vi "List Available Tags.vi"(8 "error in (no error)":errorcluster, 10 "engine":refnum<data-value>, 11 "E2E editor node in":refnum<data-value>) -> (0 "error out":errorcluster, 1 "Available Tags":refnum<class "tag descriptor.lvclass">[](array[class]), 2 "engine out":refnum<data-value>, 3 "E2E editor node out":refnum<data-value>)   [LabVIEW 2015, in "E2E Tag Exchange editor node.lvclass"]
uses:
  E2E Tag Exchange editor node.lvclass
  <vilib>/NI/DCAF/Tag Editor Core/Configuration Editor/Classes/Engine Parent/Engine Parent Editor Node.lvclass
  <vilib>/NI/Tag Bus/tag/tag descriptor.lvclass
  E2E Tag Exchange editor node.lvclass/E2E Tag Exchange editor node.ctl
  <vilib>/NI/Configuration Framework/serializable configuration/NISE_CEF_serializable configuration.lvclass/NISE_CEF_serializable configuration.ctl
  <vilib>/NI/Module Execution Interface/Engine Configuration/engine configuration.lvclass/engine configuration.ctl
  <vilib>/Utility/LVClass/Get LV Class Name.vi
  <vilib>/NI/Configuration Framework/error generator/NISE_error generator.vi
  <vilib>/NI/Module Execution Interface/Engine Configuration/engine configuration.lvclass
  <vilib>/NI/Configuration Framework/serializable configuration/NISE_CEF_serializable configuration.lvclass
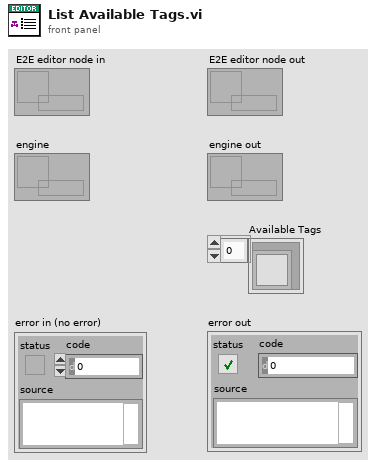
[diagram p1: front panel]
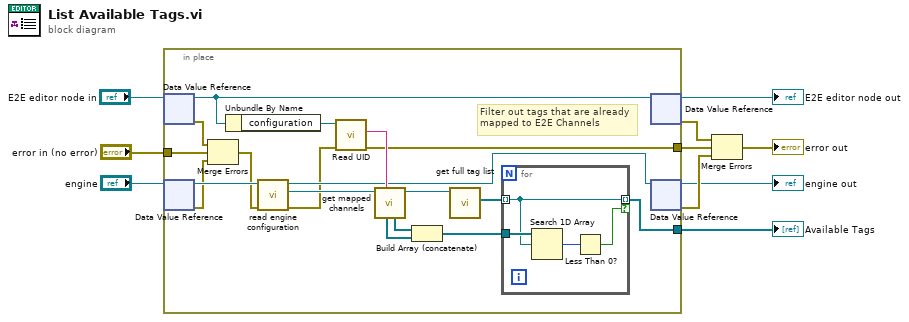
[diagram p0: block diagram]
diagram:
  n1 = in-place {
    in-place-border: "error in (no error)" -> [w15]
    in-place-border: [w17] -> w3
    in-place-border: [w11] -> w6
    # "Filter out tags that are already\nmapped to E2E Channels"
    n2 = in-place-dvr #1("E2E editor node in") -> (w19:refnum<class "E2E Tag Exchange editor node.lvclass">, w16:errorcluster)
    n3 = in-place-dvr #2("engine") -> (w28:refnum<class "Engine Parent Editor Node.lvclass">, w14:errorcluster)
    n4 = Merge Errors(w16, w15, w14) -> (w13:errorcluster)
    n5 = Unbundle By Name(w19) -> ("configuration"=w27:refnum<class "E2E Tag Exchange configuration.lvclass">)
    n6 = call <vilib>:"read engine configuration.vi"("error in"=w13, "Engine Parent Editor Node in"=w28) -> ("error out"=w12:errorcluster, "engine configuration"=w26:refnum<class "engine configuration.lvclass">, "Engine Parent Editor Node out"=w18:refnum<class "Engine Parent Editor Node.lvclass">)  [unwired: 7 in]
    n7 = call <vilib>:"Read UID.vi"("error in"=w12, "configuration in"=w27) -> ("error out"=w11:errorcluster, "instance id"=w25:string)  [unwired: 7 in, 1 out]
    n8 = call-dynamic "get mapped channels.vi"("owner"=w25, "engine configuration in"=w26) -> ("engine configuration out"=w24:refnum<class "engine configuration.lvclass">, "paired read tag"=w22:refnum<class "tag descriptor.lvclass">[], "paired write tag"=w21:refnum<class "tag descriptor.lvclass">[])  [unwired: 5 in, 2 out]
    n9 = Build Array (concatenate)(w22, w21) -> (w20:refnum<class "tag descriptor.lvclass">[])
    n10 = call <vilib>:"get full tag list.vi"("engine configuration in"=w24) -> ("tag list"=w23:refnum<class "tag descriptor.lvclass">[])  [unwired: 9 in, 1 out]
    n11 = for {
      tunnel: w23 -> [w31] mode=indexing
      tunnel: w20 -> [w32]
      tunnel: [w31] -> w17 mode=indexing if=w29
      n12 = Search 1D Array(1D array=w32, element=w31) -> (index of element=w30:i32)  [unwired: 1 in]
      n13 = Less Than 0?(x=w30) -> (x < 0?=w29:bool)
    }
    n14 = in-place-dvr #1(w19) -> (→"E2E editor node out":refnum<data-value>, w7:errorcluster)
    n15 = in-place-dvr #2(w18) -> (→"engine out":refnum<data-value>, w5:errorcluster)
  }
  "Available Tags" <- w3
  n16 = Merge Errors(w7, w6, w5) -> (→"error out":errorcluster)
